vi "VCS Get Velocity Units.vi"(0 "axis in":cluster{"keyHandle":u32, "nodeId":u16}={"keyHandle"=0, "nodeId"=1}, 11 "error in (no error)":errorcluster) -> (4 "axis out":cluster{"keyHandle":u32, "nodeId":u16}={"keyHandle"=0, "nodeId"=1}, 6 "index":T1={"velocity dimension"=164, "velocity notation"=0} {"velocity dimension" items=["revolution / time (rev/time)"=164]; "velocity notation" items=["standard"=0, "deci"=-1, "centi"=-2, "milli"=-3]}, 15 "error out":errorcluster)   [LabVIEW 2010]
doc: "<B>VCS_GetVelocityUnits</B> reads velocity unit parameters."
uses:
  Resources/EposCmd.dll
  Resources/EposCmd64.dll
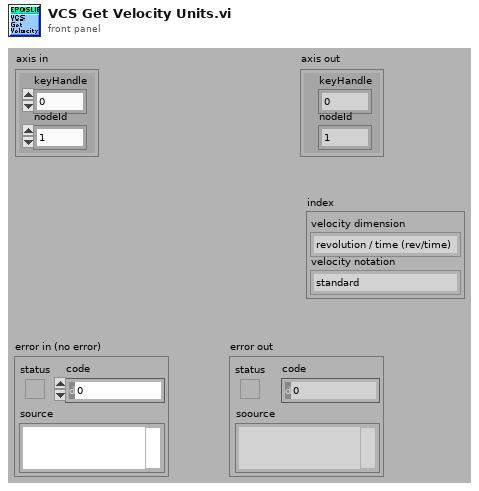
[diagram p1: front panel]
types:
  T1 = cluster{"velocity dimension":u8, "velocity notation":i8}
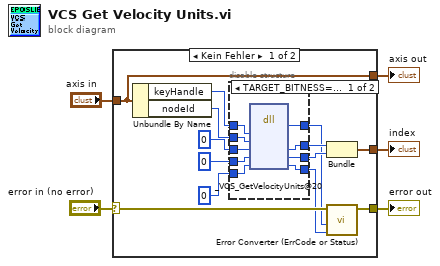
[diagram p0: block diagram]
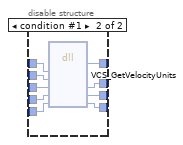
[diagram p2: hidden frame]
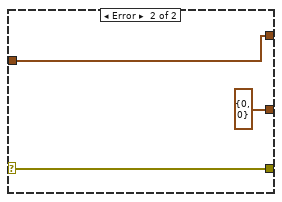
[diagram p3: hidden frame]
diagram:
  n1 = case shown="Kein Fehler" "error in (no error)" {
    selector: "error in (no error)" -> [w16 w38]
    tunnel: "axis in" -> [w18 w39]
    tunnel: [w18 w39] -> w4
    tunnel: [w17 w38] -> w3
    tunnel: [w8 cluster{"pVelDimension":u8, "pVelNotation":i8} {"pVelDimension"=0, "pVelNotation"=0}] -> w1
    frame No Error {
      n2 = Unbundle By Name(w18) -> ("keyHandle"=w14:u32, "nodeId"=w13:u16)
      n3 = disable-structure shown="TARGET_BITNESS==32, Standard" {
        disable-tunnel: u32 0 ("pErrorCode") -> [w27 w36]
        disable-tunnel: w14 -> [w26 w35]
        disable-tunnel: w13 -> [w25 w34]
        disable-tunnel: u8 0 ("pVelDimension") -> [w24 w33]
        disable-tunnel: [w23 w32] -> w11
        disable-tunnel: [w22 w31] -> w10
        disable-tunnel: i8 0 ("pVelNotation") -> [w21 w30]
        disable-tunnel: [w20 w29] -> w7
        disable-tunnel: [w19 w28] -> w6
        frame condition #0 (active) {
          n4 = dll-call lib="C:/Sources/LabView/maxon EPOS/Resources/EposCmd.*" fn="_VCS_GetVelocityUnits@20"("KeyHandle"=w26, "NodeId"=w25, "pVelDimension"=w24, "pVelNotation"=w21, "pErrorCode"=w27) -> ("Rückgabetyp"=w20:i32, "pVelDimension"=w23:u8, "pVelNotation"=w22:i8, "pErrorCode"=w19:u32)  [unwired: 5 in, 2 out]
        }
        frame condition #1 {
          n5 = dll-call lib="C:/setup/Resources/EposCmd64.*" fn="VCS_GetVelocityUnits" ("EposCmd.dll:_VCS_GetVelocityUnits@20")("KeyHandle"=w35, "NodeId"=w34, "pVelDimension"=w33, "pVelNotation"=w30, "pErrorCode"=w36) -> ("Rückgabetyp"=w29:i32, "pVelDimension"=w32:u8, "pVelNotation"=w31:i8, "pErrorCode"=w28:u32)  [unwired: 5 in, 2 out]
        }
      }
      n6 = Bundle("pVelDimension"=w11, "pVelNotation"=w10) -> (w8:cluster{"pVelDimension":u8, "pVelNotation":i8})  [unwired: 1 in]
      n7 = call "Error Converter (ErrCode or Status).vi"("error code"=w6, "return type"=w7, "error in (no error)"=w16) -> ("error out"=w17:errorcluster)  [unwired: 7 in]
    }
    frame Error {
    }
  }
  "error out" <- w3
  "axis out" <- w4
  "index" <- w1
